vi "getNodeIdMote.vi"(1 "input data":string) -> (0 "node id (1 byte)":u8)   [LabVIEW 2011]
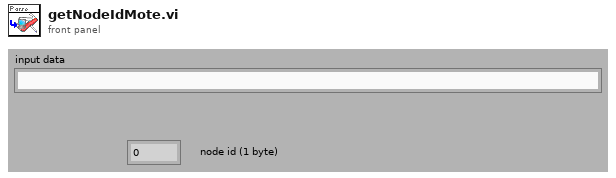
[diagram p1: front panel]
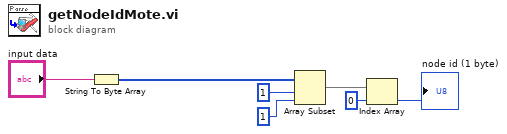
[diagram p0: block diagram]
diagram:
  n1 = String To Byte Array(string="input data") -> (unsigned byte array=w1:u8[])
  n2 = Array Subset(array=w1, index=1 ("x"), length=1 ("x")) -> (w3:u8[])
  n3 = Index Array(array=w3, index=0) -> (element=→"node id (1 byte)":u8)
